vi "Create Temporary Duplicate Project.vi"(8 "error in":errorcluster, 11 "project path":path) -> (0 "error out":errorcluster, 3 "temp project path":path)   [LabVIEW 2020, in "Template Tool.lvlib"]
uses:
  Template Tool.lvlib
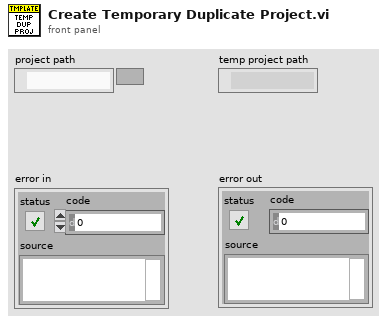
[diagram p1: front panel]
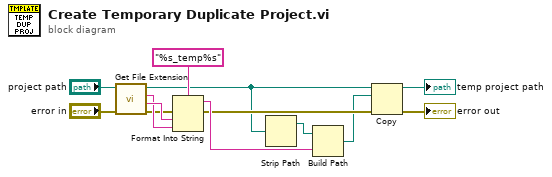
[diagram p0: block diagram]
diagram:
  n1 = call <vilib>:"Get File Extension.vi"("error in (no error)"="error in", "file"="project path") -> ("error out"=w10:errorcluster, "filename without extension"=w12:string, "lowercase file extension"=w11:string, "dup file"=w1:path)  [unwired: 5 in, 1 out]
  n2 = Format Into String(format string="%s_temp%s", error in=w10, w12, w11) -> (resulting string=w8:string, error out=w5:errorcluster)  [unwired: 1 in]
  n3 = Strip Path(path=w1) -> (stripped path=w9:path)  [unwired: 1 out]
  n4 = Build Path(base path=w9, name or relative path=w8) -> (appended path=w4:path)
  n5 = Copy(8:w5, 10:w4, 11:w1) -> (0:→"error out":errorcluster, 3:→"temp project path":path)  [unwired: 2 in, 1 out]
